vi "Graphics-Create Intensity Color Map.vi"() -> (0 "Array":cluster{dbl, "Color":u32}[](array[cluster]))   [LabVIEW 2020]
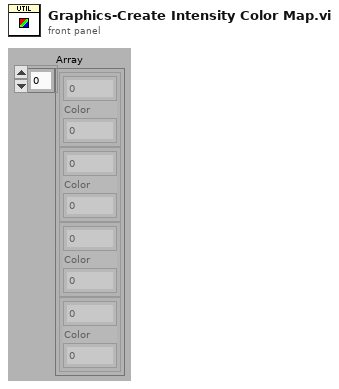
[diagram p1: front panel]
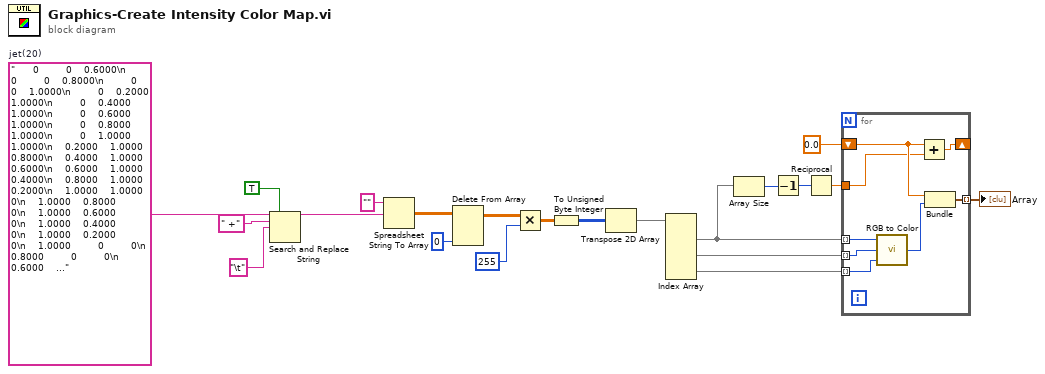
[diagram p0: block diagram]
diagram:
  w21 = "      0         0    0.6000\n         0         0    0.8000\n         0         0    1.0000\n         0    0.2000    1.0000\n         0    0.4000    1.0000\n         0    0.6000    1.0000\n         0    0.8000    1.0000\n         0    1.0000    1.0000\n    0.2000    1.0000    0.8000\n    0.4000    1.0000    0.6000\n    0.6000    1.0000    0.4000\n    0.8000    1.0000    0.2000\n    1.0000    1.0000         0\n    1.0000    0.8000         0\n    1.0000    0.6000         0\n    1.0000    0.4000         0\n    1.0000    0.2000         0\n    1.0000         0         0\n    0.8000         0         0\n    0.6000         0         0"  # jet(20)
  n1 = Search and Replace String(replace all?=TRUE ("replace all? (F)"), input string=w21, search string=" +", replace string="\t" ("replace string (\"\")")) -> (result string=w17:string)  [unwired: 4 in, 3 out]
  n2 = Spreadsheet String To Array(format string="", spreadsheet string=w17) -> (array=w15:dbl[][])  [unwired: 2 in]
  n3 = Delete From Array(array=w15, index (col)=0 ("disabled index (col)")) -> (array with subset deleted=w13:dbl[][])  [unwired: 2 in, 1 out]
  n4 = Multiply(x=w13, y=u8 255) -> (x*y=w11:dbl[][])
  n5 = To Unsigned Byte Integer(number=w11) -> (unsigned 8bit integer=w10:u8[][])
  n6 = Transpose 2D Array(2D array=w10) -> (transposed array=w1:u8[][])
  n7 = Index Array(array=w1) -> (element #1=w7:u8[], element #2=w9:u8[], element #3=w8:u8[])  [unwired: 6 in]
  n8 = Array Size(array=w7) -> (size(s)=w3:i32)
  n9 = Decrement(x=w3) -> (x-1=w5:i32)
  n10 = Reciprocal(x=w5) -> (1/x=w4:dbl)
  n11 = for {
    tunnel: w7 -> [w29] mode=indexing
    tunnel: w9 -> [w28] mode=indexing
    tunnel: w8 -> [w27] mode=indexing
    shift-right: [w24] -> _
    shift-left: 0.0 -> [w23]
    tunnel: w4 -> [w22]
    tunnel: [w25] -> w2 mode=indexing
    n12 = call <vilib>:"RGB to Color.vi"("B"=w27, "G"=w28, "R"=w29) -> ("Color"=w26:u32)
    n13 = Add(x=w23, y=w22) -> (x+y=w24:dbl)
    n14 = Bundle(w23, "Color"=w26) -> (w25:cluster{dbl, "Color":u32})  [unwired: 1 in]
  }
  "Array" <- w2
